vi "Gen_Square_0to10V.vi"(5 "reset signal":bool, 6 "sampling info":cluster{"Fs":dbl, "#s":dbl}={"Fs"=500000.0, "#s"=100000.0} {"Fs" format="%.2p"}, 8 "error in (no error)":errorcluster, 9 "Width (ms)":dbl=0.1 format="%0.2f", 10 "amplitude":dbl format="%0.2p", 11 "frequency":dbl=1.0 format="%0.2p") -> (0 "error out":errorcluster, 1 "signal out":waveform(dbl)={"t0"=timestamp(6.999999999999999 s since 1904-01-01), "dt"=2e-06, "Y"=array[100000 elements]})   [LabVIEW 2012]
uses:
  <vilib>/measure/maUtilsandCtls.llb/ma_Updatet0 timestamp.vi
  <vilib>/measure/NI_MABase.lvlib
  <vilib>/Analysis/NI_AALBase.lvlib
panel:
  out "phase out":dbl=62.0 format="%.2p"
  in  "phase":dbl=340.0 format="%.2p"
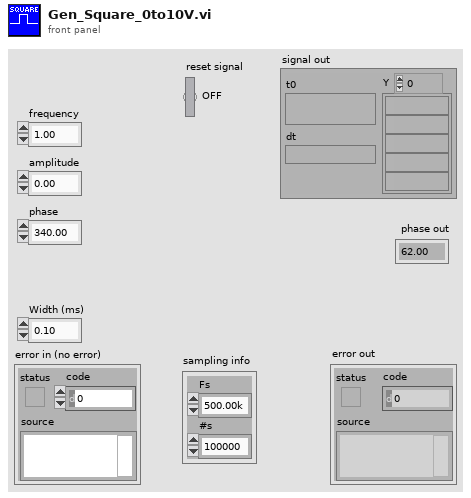
[diagram p1: front panel]
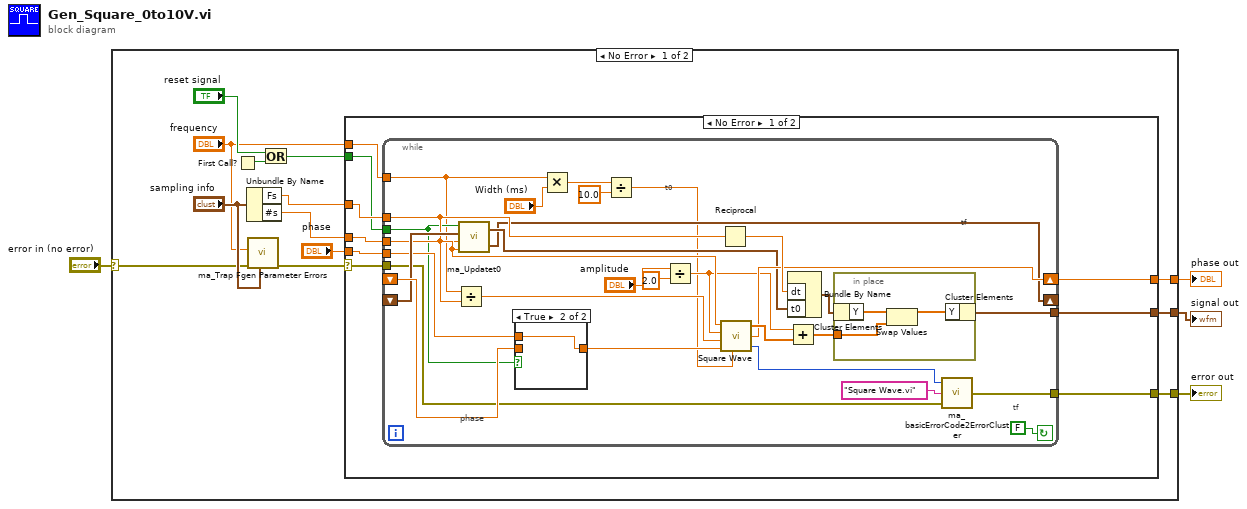
[diagram p0: block diagram]
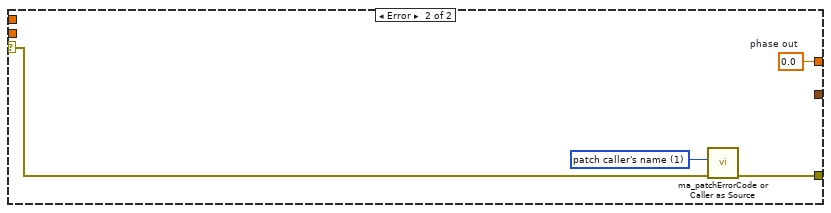
[diagram p3: hidden frame]
diagram:
  n1 = case shown="No Error" "error in (no error)" {
    selector: "error in (no error)" -> [w8 w65]
    tunnel: [w17 w65] -> w4
    tunnel: [w6 _] -> w2
    tunnel: [w5 _] -> w1
    frame No Error {
      n2 = First Call?() -> (First Call?: T/F=w11:bool)
      n3 = Unbundle By Name("sampling info") -> ("Fs"=w13:dbl, "#s"=w12:dbl)
      n4 = call <vilib>:"ma_Trap Fgen Parameter Errors.vi"("Sampling info"="sampling info", "error in (no error)"=w8, "frequency"="frequency") -> ("error out"=w16:errorcluster)  [unwired: 8 in]
      n5 = Or(x="reset signal", y=w11) -> (x .or. y?=w9:bool)
      n6 = case shown="No Error" w16 {
        selector: w16 -> [w20 w63]
        tunnel: [w26 w64] -> w5
        tunnel: [w25 w62] -> w17
        tunnel: "phase" -> [w24 _]
        tunnel: w13 -> [w23 _]
        tunnel: w12 -> [w22 _]
        tunnel: w9 -> [w21 _]
        tunnel: [w18 _] -> w6
        tunnel: "frequency" -> [w19 _]
        frame No Error {
          n7 = while {
            tunnel: w20 -> [w41]
            tunnel: w21 -> [w44]
            tunnel: w22 -> [w46]
            tunnel: w23 -> [w45]
            tunnel: w24 -> [w53]
            tunnel: [w40] -> w25
            shift-left: _ -> [w55]
            shift-right: [w47] -> w26
            shift-left: _ -> [w54]
            shift-right: [w37] -> _
            tunnel: w19 -> [w30]
            tunnel: [w35] -> w18
            stop <- FALSE continue-if-true
            # "tf"
            # "t0"
            # "phase"
            # "tf"
            n8 = Divide(x=w30, y=w45) -> (x/y=w50:dbl)
            n9 = call-poly <vilib>:"ma_Updatet0.vi"("samples"=w46, "sampling rate (S/s)"=w45, "tf previous"=w54, "Reset Generation"=w44) -> ("tf new"=w37:timestamp, "t0"=w39:timestamp)
            n10 = case shown="True" w44 {
              tunnel: w55 -> [w59 _]
              tunnel: [w59 w60] -> w48
              tunnel: w53 -> [_ w60]
              frame False {
              }
              frame True {
              }
            }
            n11 = Multiply(x=w30, y="Width (ms)") -> (x*y=w29:dbl)
            n12 = Divide(x=w29, y=10.0) -> (x/y=w28:dbl)
            n13 = Divide(x="amplitude", y=2.0) -> (x/y=w32:dbl)
            n14 = Reciprocal(x=w45) -> (1/x=w51:dbl)
            n15 = call <vilib>:"Square Wave.vi"("samples"=w46, "amplitude"=w32, "frequency"=w50, "duty cycle (%)"=w28, "phase in"=w48) -> ("square wave"=w49:dbl[], "phase out"=w47:dbl, "error"=w42:i32)  [unwired: 1 in]
            n16 = Bundle By Name("dt"=w51, "t0"=w39) -> (w36:waveform(dbl))  [unwired: 1 in]
            n17 = Add(x=w32, y=w49) -> (x+y=w38:dbl[])
            n18 = in-place {
              in-place-border: w38 -> [w56]
              n19 = in-place-cluster #1(w36) -> ("Y"=w58:dbl[])
              n20 = Swap Values(12:w58, 14:w56) -> (1:w57:dbl[])  [unwired: 1 in, 1 out]
              n21 = in-place-cluster #1("Y"=w57) -> (w35:waveform(dbl))
            }
            n22 = call <vilib>:"ma_basicErrorCode2ErrorCluster.vi"("error in (no error)"=w41, "subVI name"="Square Wave.vi" ("subVI Name"), "Error Code"=w42) -> ("error out"=w40:errorcluster)
          }
        }
        frame Error {
          w61 = u16 1 items=["patch error code", "patch caller's name"] ("operation")
          w64 = 0.0  # phase out
          n23 = call <vilib>:"ma_patchErrorCode or Caller as Source.vi"("error in (no error)"=w63, "operation"=w61) -> ("error out"=w62:errorcluster)  [unwired: 9 in]
        }
      }
    }
    frame Error {
    }
  }
  "error out" <- w4
  "signal out" <- w2
  "phase out" <- w1
